vi "Autonomous Independent.vi"() -> ()   [LabVIEW 2012]
doc: "This VI is called when autonomous begins, and will automatically be terminated when autonomous ends. You can carry out timed or sensor driven robot movement independently without needing to return to the caller."
uses:
  AutoInstruction.ctl
  AutoEnum.ctl
  Robot Global Data.vi
  <vilib>/Rock Robotics/WPI/RobotDrive/WPI_RobotDriveArcadeDrive_Standard(NoSaturation).vi
panel:
  in  "Instructions":T1(array[cluster])
  in  "Instruction Sequence":T2(array[cluster])
  in  "AutoInstruction":T3
  in  "Default":T3[](array[typedef])
  in  "BackRight":T3[](array[typedef])
  in  "BackLeft":T3[](array[typedef])
  in  "FrontRight":T3[](array[typedef])
  in  "FrontLeft":T3[](array[typedef])
  out "AutoEnum":u16
  out "Current Movement, for debugging":T4 {"Y Joystick Value" scale=1.0..-1.0; "X Joystick Value" scale=-1.0..1.0}
  in  "Array of robot movements":T5(array[cluster]) {"Y Joystick Value" scale=1.0..-1.0; "X Joystick Value" scale=-1.0..1.0}
  # "Be sure to right-click and choose Data Operations>>Make Current Value default if you want to save the array values with the VI"
  # "REMEMBER TO SET AS DEFAULT"
  # "GLENN'S STUFF"
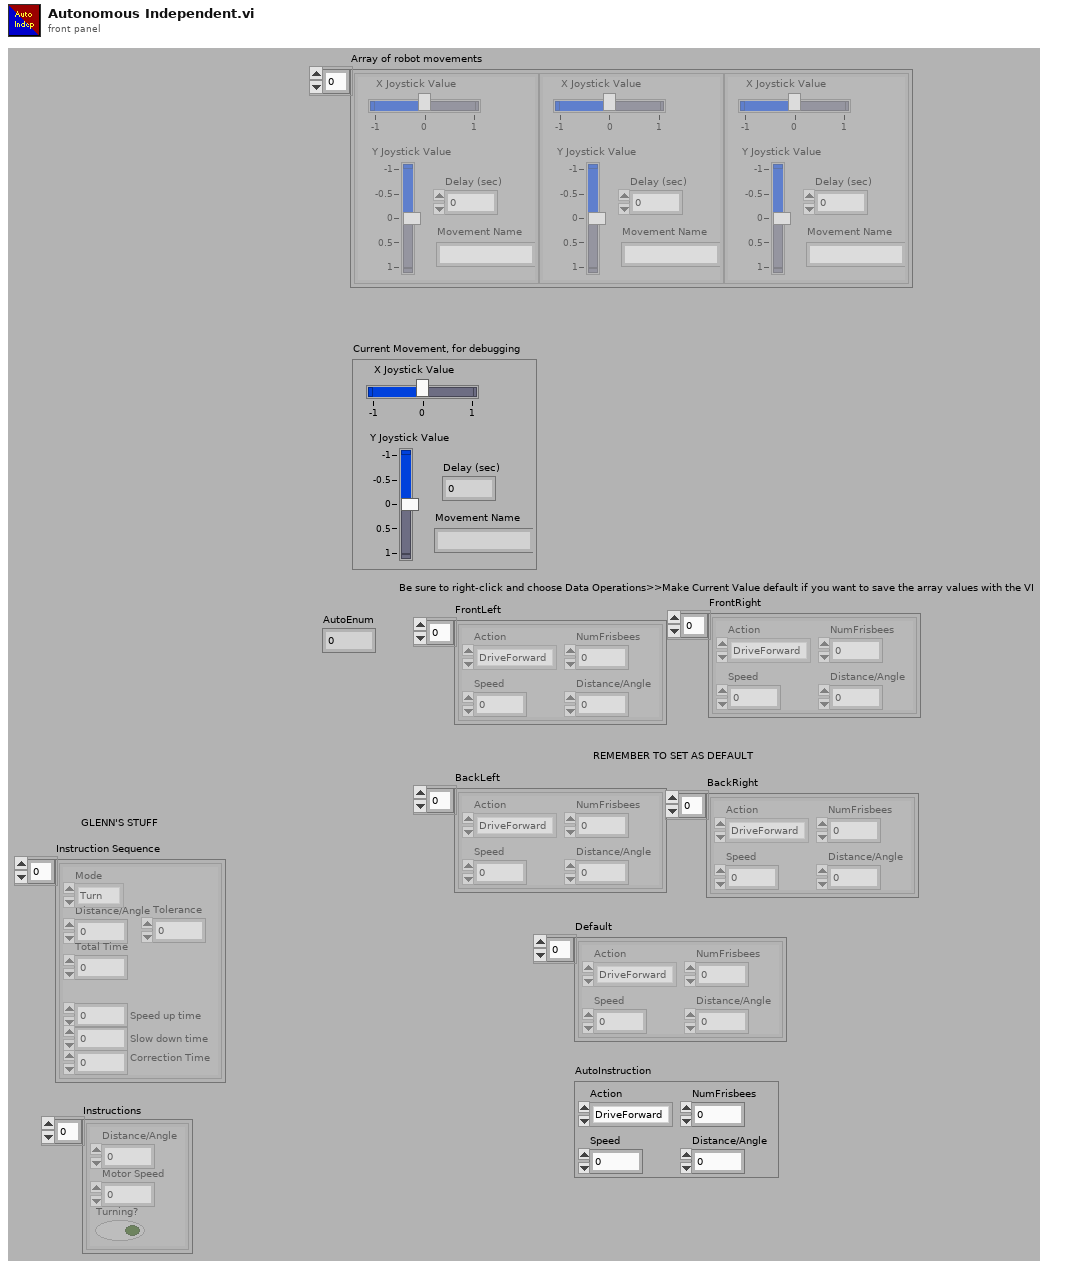
[diagram p1: front panel]
types:
  T1 = cluster{"Distance/Angle":dbl, "Motor Speed":dbl, "Turning?":bool}[]
  T2 = cluster{"Distance/Angle":dbl, "Tolerance":dbl, "Total Time":dbl, "Mode":enum16{"Turn", "Drive"}, "Correction Time":dbl, "Speed up time":dbl, "Slow down time":dbl}[]
  T3 = typedef "AutoInstruction.ctl" = cluster{"Distance/Angle":dbl, "Speed":dbl, "Action":enum16{"DriveForward", "Turn", "Aim", "Shoot"}, "NumFrisbees":i32}
  T4 = cluster{"X Joystick Value":dbl, "Y Joystick Value":dbl, "Delay (sec)":dbl, "Movement Name":string}
  T5 = cluster{"X Joystick Value":dbl, "Y Joystick Value":dbl, "Delay (sec)":dbl, "Movement Name":string}[]
  T6 = typedef "AutoEnum.ctl" = enum16{"Disabled", "BackRight", "BackLeft", "CloseRight", "CloseLeft"}
  T7 = typedef "WPI_EncoderDevRef.ctl" = cluster{"DevStatus":errorcluster, "EncoderIndex":T8, "CounterIndex":T9, "DistancePerCount":dbl, "Decoding Type":T10}
  T8 = typedef "FPGA_EncoderIdx.ctl" = enum8{"Enc 0", "Enc 1", "Enc 2", "Enc 3", "Invalid"}
  T9 = typedef "FPGA_CounterCtrSystemIndex.ctl" = enum8{"Ctr 0", "Ctr 1", "Ctr 2", "Ctr 3", "Ctr 4", "Ctr 5", "Ctr 6", "Ctr 7", "Invalid"}
  T10 = typedef "WPI_EncoderType.ctl" = enum16{"1x", "2x", "4x"}
  T11 = typedef "WPI_JoystickDevRef.ctl" = cluster{"Device":T12}
  T12 = typedef "WPI_JoystickDeviceEnum.ctl" = enum16{"USB 1", "USB 2", "USB 3", "USB 4", "Kinect 1", "Kinect 2"}
  T13 = cluster{"axis 1 (x)":dbl, "axis 2 (y)":dbl, "axis 3 (throttle)":dbl, "axis 4":dbl, "axis 5":dbl, "axis 6":dbl}
  T14 = typedef "WPI_GyroDevRef.ctl" = cluster{"DevStatus":errorcluster, "Analog Module":T15, "Analog Channel":T16, "Offset":dbl, "Gain (VoltsPerDegree/Second)":dbl}
  T15 = typedef "FPGA_TypedefAnalogModule.ctl" = enum16{"Analog Module 1", "Analog Module 2"}
  T16 = typedef "FPGA_AIChannel.ctl" = enum8{"AI 1", "AI 2", "AI 3", "AI 4", "AI 5", "AI 6", "AI 7", "AI 8", "Invalid"}
  T17 = typedef "WPI_RobotDriveDevRef.ctl" = cluster{"DevStatus":errorcluster, "Motors[]":T18[], "Square Inputs":bool, "Max Output":dbl, "Isochronous":bool}
  T18 = typedef "WPI_MotorControlDeviceRef.ctl" = cluster{"DeviceStatus":errorcluster, "Type":enum16{"PWM", "CAN"}, "PWM":cluster{"Digital Module":T19, "PWM Channel":T20, "DeadBand":T21}, "CAN":cluster{"Device Number":u8, "Control Mode":T22, "Semaphore":T23, "Max Vout":dbl}, "Invert":bool, "TransformRef":T24, "InvTransformRef":T24}
  T19 = typedef "FPGA_TypedefDigitalModule.ctl" = enum16{"Digital Module 1", "Digital Module 2"}
  T20 = typedef "FPGA_DIOPWMChannel.ctl" = enum8{"PWM 1", "PWM 2", "PWM 3", "PWM 4", "PWM 5", "PWM 6", "PWM 7", "PWM 8", "PWM 9", "PWM 10", "Invalid"}
  T21 = typedef "WPI_PWMDeadband.ctl" = cluster{"Name":string, "maxPositivePwm":i32, "minPositivePwm":i32, "centerPwm":i32, "maxNegativePwm":i32, "minNegativePwm":i32, "angularRange":u16}
  T22 = typedef "WPI_CANJaguar_ControlMode.ctl" = enum8{"Percent VBus", "Current", "Speed", "Position", "Voltage"}
  T23 = typedef "Semaphore RefNum" = refnum<k1>
  T24 = typedef "WPI_PWMTransform_ConPane.ctl" = refnum<vi>
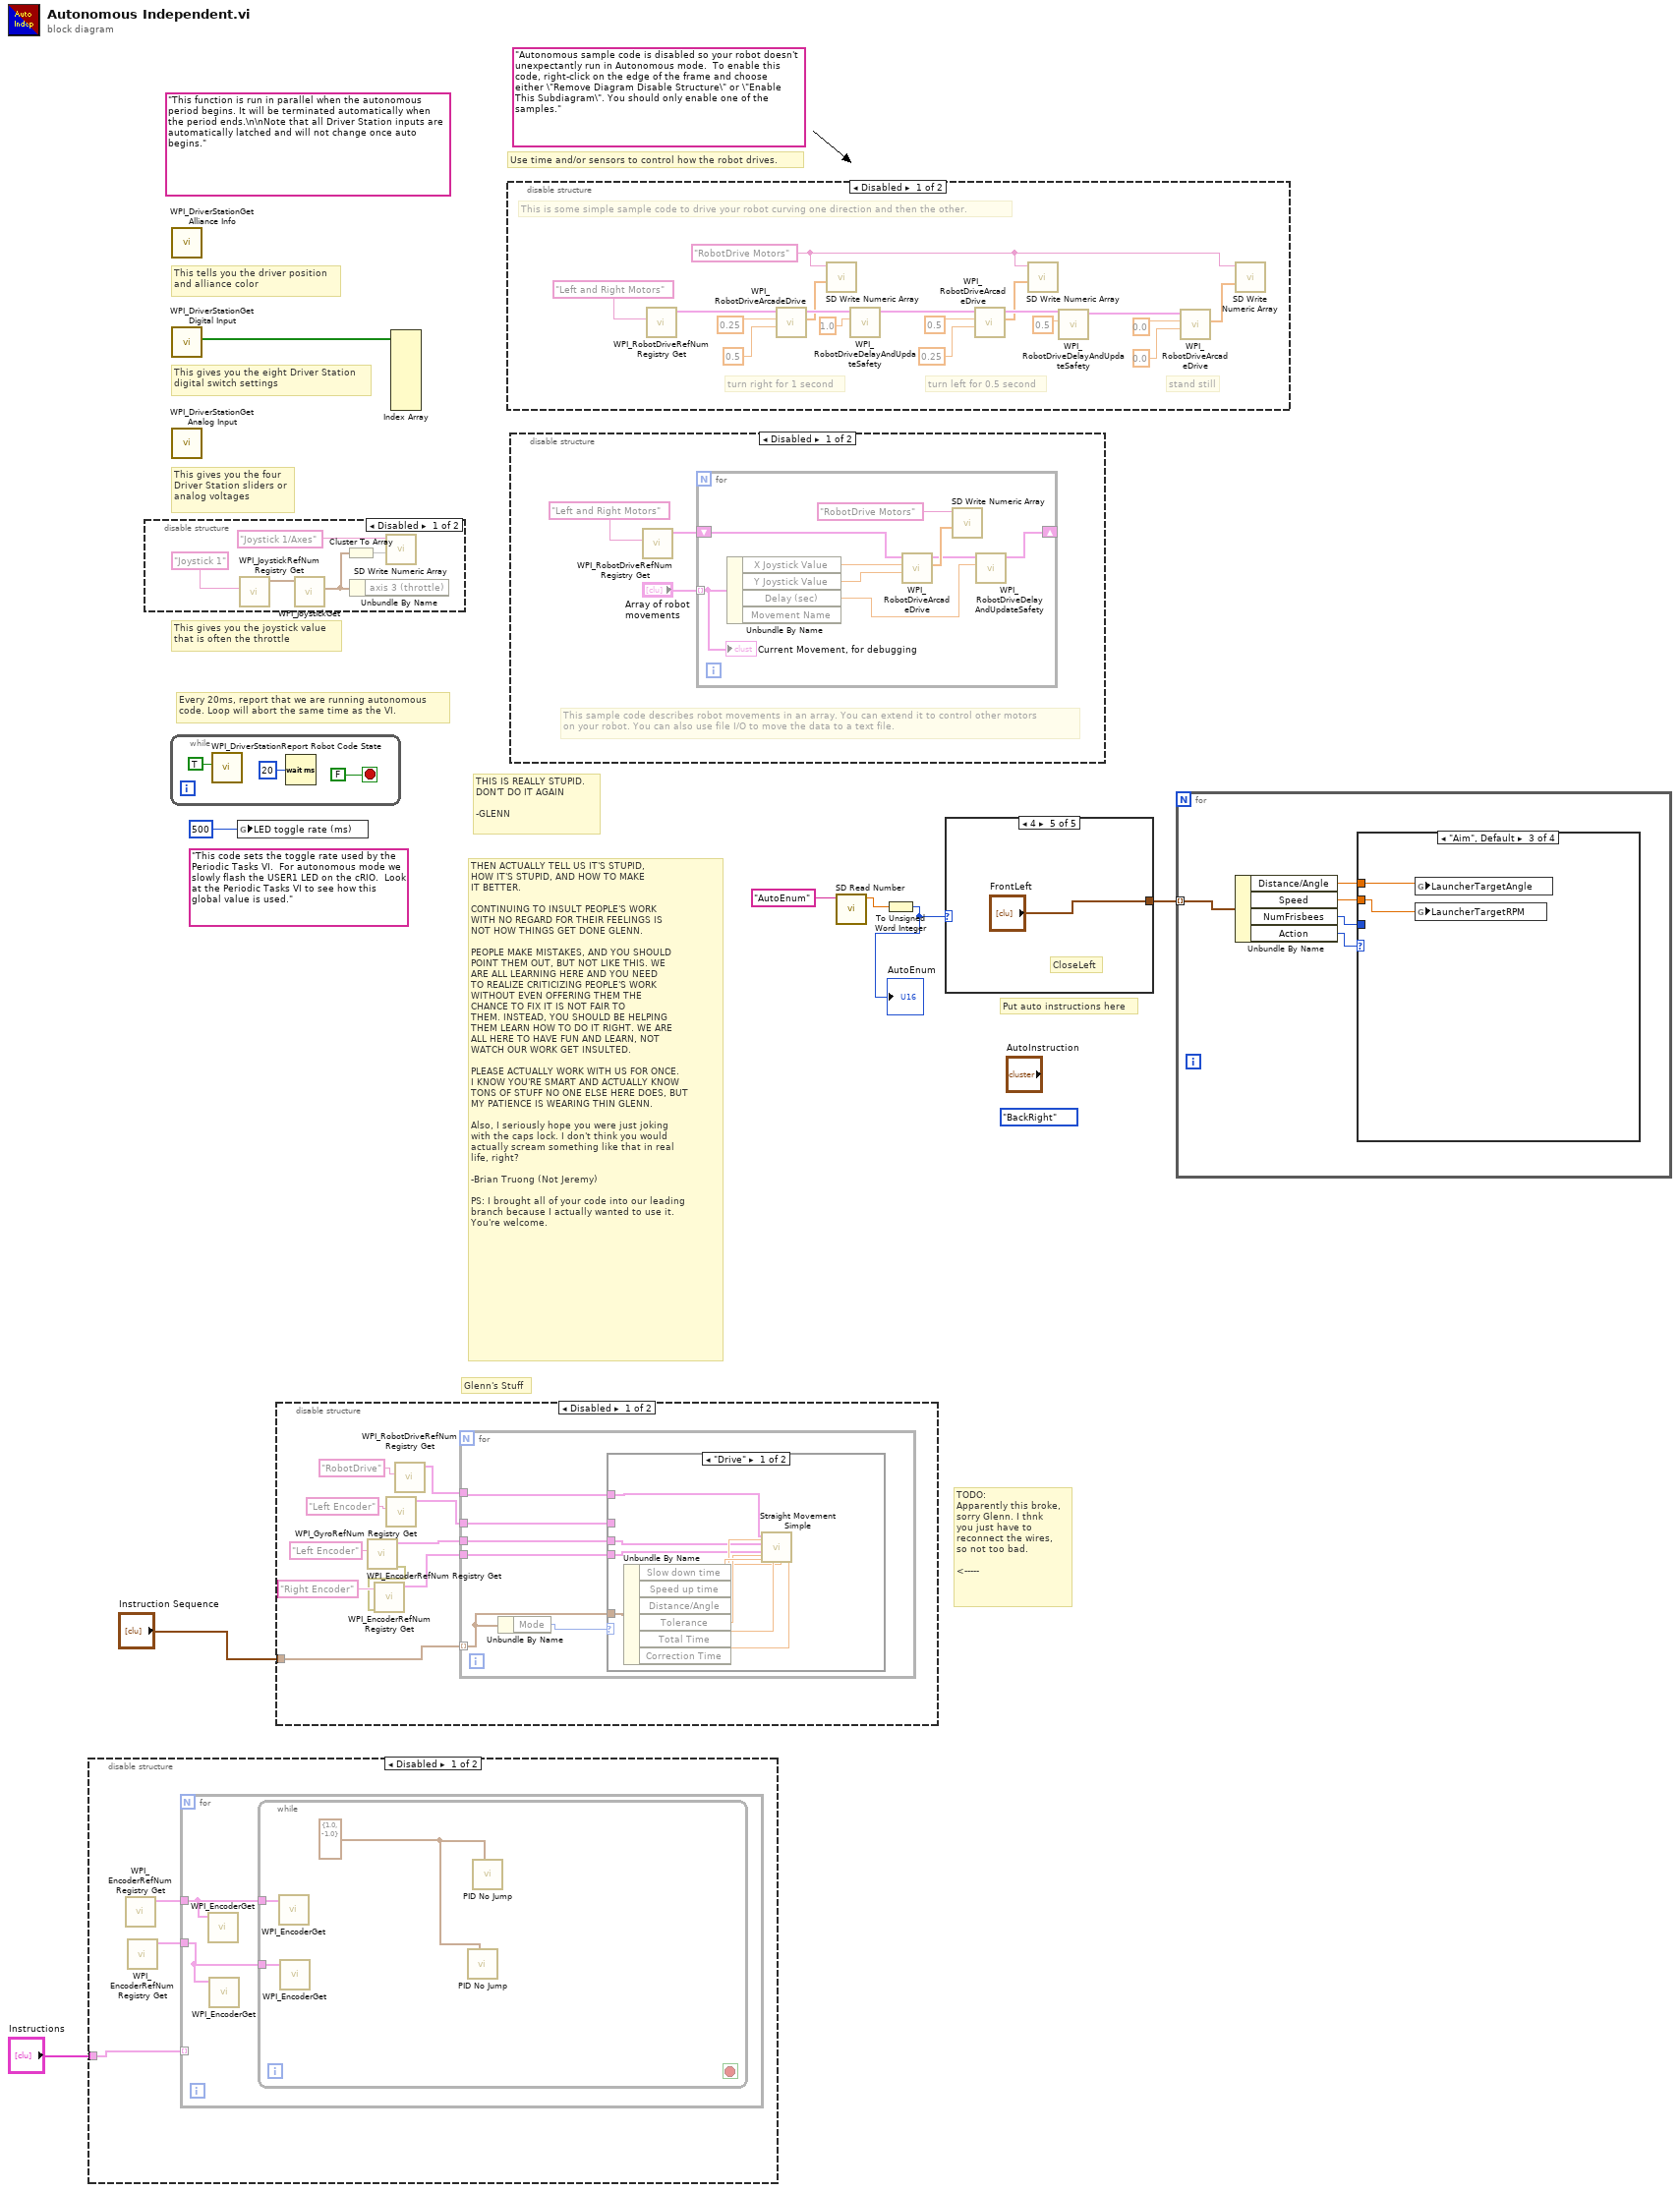
[diagram p0: block diagram]
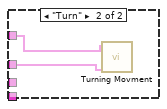
[diagram p4: hidden frame]
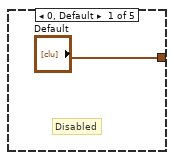
[diagram p6: hidden frame]
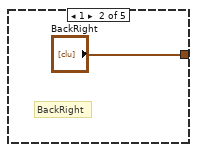
[diagram p7: hidden frame]
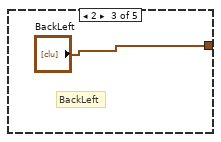
[diagram p8: hidden frame]
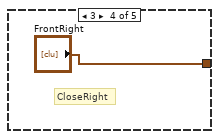
[diagram p9: hidden frame]
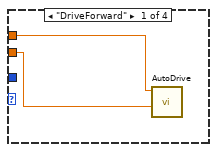
[diagram p10: hidden frame]
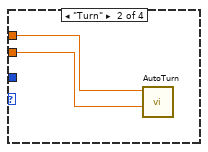
[diagram p11: hidden frame]
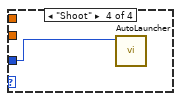
[diagram p12: hidden frame]
diagram:
  (unwired) AutoEnum."BackRight" ("AutoEnum")
  (unwired) "This code sets the toggle rate used by the Periodic Tasks VI.  For autonomous mode we slowly flash the USER1 LED on the cRIO.  Look at the Periodic Tasks VI to see how this global value is used."
  (unwired) "Autonomous sample code is disabled so your robot doesn't unexpectantly run in Autonomous mode.  To enable this code, right-click on the edge of the frame and choose either \"Remove Diagram Disable Structure\" or \"Enable This Subdiagram\". You should only enable one of the samples."
  (unwired) "This function is run in parallel when the autonomous period begins. It will be terminated automatically when the period ends.\n\nNote that all Driver Station inputs are automatically latched and will not change once auto begins."
  # "TODO:\nApparently this broke,\nsorry Glenn. I thnk\nyou just have to\nreconnect the wires,\nso not too bad.\n\n<-----"
  # "Glenn's Stuff"
  # "THEN ACTUALLY TELL US IT'S STUPID,\nHOW IT'S STUPID, AND HOW TO MAKE\nIT BETTER.\n\nCONTINUING TO INSULT PEOPLE'S WORK\nWITH NO REGARD FOR THEIR FEELINGS IS\nNOT HOW THINGS GET DONE GLENN.\n\nPEOPLE MAKE MISTAKES, AND YOU SHOULD\nPOINT THEM OUT, BUT NOT LIKE THIS. WE\nARE ALL LEARNING HERE AND YOU NEED\nTO REALIZE CRITICIZING PEOPLE'S WORK\nWITHOUT EVEN OFFERING THEM THE\nCHANCE TO FIX IT IS NOT FAIR TO\nTHEM. INSTEAD, YOU SHOULD BE HELPING\nTHEM LEARN HOW TO DO IT RIGHT. WE ARE\nALL HERE TO HAVE FUN AND LEARN, NOT\nWATCH OUR WORK GET INSULTED.\n\nPLEASE ACTUALLY WORK WITH US FOR ONCE.\nI KNOW YOU'RE SMART AND ACTUALLY KNOW\nTONS OF STUFF NO ONE ELSE HERE DOES, BUT\nMY PATIENCE IS WEARING THIN GLENN.\n\nAlso, I seriously hope you were just joking\nwith the caps lock. I don't think you would\nactually scream something like that in real\nlife, right?\n\n-Brian Truong (Not Jeremy)\n\nPS: I brought all of your code into our leading\nbranch because I actually wanted to use it.\nYou're welcome."
  # "THIS IS REALLY STUPID.\nDON'T DO IT AGAIN\n\n-GLENN"
  # "Put auto instructions here"
  # "Every 20ms, report that we are running autonomous\ncode. Loop will abort the same time as the VI."
  # "This gives you the joystick value\nthat is often the throttle"
  # "Use time and/or sensors to control how the robot drives."
  # "This tells you the driver position\nand alliance color"
  # "This gives you the eight Driver Station\ndigital switch settings"
  # "This gives you the four\nDriver Station sliders or\nanalog voltages"
  n1 = disable-structure shown="Disabled" {
    disable-tunnel: "Instructions" -> [w9 _]
    frame Disabled {
      n2 = call <vilib>:"WPI_EncoderRefNum Registry Get.vi"() -> ("EncoderDevRef"=w11:T7)  [unwired: 10 in, 1 out]
      n3 = call <vilib>:"WPI_EncoderRefNum Registry Get.vi"() -> ("EncoderDevRef"=w10:T7)  [unwired: 10 in, 1 out]
      n4 = for {
        tunnel: w11 -> [w13]
        tunnel: w10 -> [w12]
        tunnel: w9 -> [_] mode=indexing
        n5 = call <vilib>:"WPI_EncoderGet.vi"("EncoderDevRef"=w13) -> ()  [unwired: 5 in, 6 out]
        n6 = call <vilib>:"WPI_EncoderGet.vi"("EncoderDevRef"=w12) -> ()  [unwired: 5 in, 6 out]
        n7 = while {
          tunnel: w13 -> [w15]
          tunnel: w12 -> [w16]
          stop <- _ stop-if-true
          w14 = cluster{"output high":dbl, "output low":dbl} {"output high"=1.0, "output low"=-1.0} ("output range")
          n8 = call <vilib>:"WPI_EncoderGet.vi"("EncoderDevRef"=w15) -> ()  [unwired: 5 in, 6 out]
          n9 = call <vilib>:"WPI_EncoderGet.vi"("EncoderDevRef"=w16) -> ()  [unwired: 5 in, 6 out]
          n10 = call "PID No Jump.vi"("output range"=w14) -> ()  [unwired: 10 in, 1 out]
          n11 = call "PID No Jump.vi"("output range"=w14) -> ()  [unwired: 10 in, 1 out]
        }
      }
    }
    frame Enabled {
    }
  }
  n12 = disable-structure shown="Disabled" {
    frame Disabled {
      n13 = call <vilib>:"WPI_JoystickRefNum Registry Get.vi"("refnum name"="Joystick 1") -> ("JoystickDevRef"=w20:T11)  [unwired: 1 in, 9 out]
      n14 = call <vilib>:"WPI_JoystickGet.vi"("JoystickDevRef"=w20) -> ("Axes"=w18:T13)  [unwired: 1 in, 5 out]
      n15 = Cluster To Array(cluster=w18) -> (array=w19:dbl[])
      n16 = Unbundle By Name(w18) -> ()  [unwired: 1 out]
      n17 = call <vilib>:"SD Write Numeric Array.vi"("Numeric Array"=w19, "Name"="Joystick 1/Axes") -> ()  [unwired: 8 in, 2 out]
    }
    frame Enabled {
    }
  }
  n18 = while {
    stop <- FALSE stop-if-true
    n19 = call <vilib>:"WPI_DriverStationReport Robot Code State.vi"("Autonomous"=TRUE) -> ()  [unwired: 10 in, 1 out]
    n20 = Wait (ms)(milliseconds to wait=u32 20) -> ()  [unwired: 1 out]
  }
  n21 = call <vilib>:"WPI_DriverStationGet Alliance Info.vi"() -> ()  [unwired: 12 out]
  n22 = call <vilib>:"WPI_DriverStationGet Digital Input.vi"() -> ("Driver Station Digital Input (1-8)"=w8:bool[])  [unwired: 11 out]
  n23 = call <vilib>:"WPI_DriverStationGet Analog Input.vi"() -> ()  [unwired: 12 out]
  n24 = global write "Robot Global Data.vi" "LED toggle rate (ms)"(u32 500 ("LED ms toggle rate")) -> ()
  n25 = disable-structure shown="Disabled" {
    disable-tunnel: "Instruction Sequence" -> [w34 _]
    frame Disabled {
      n26 = call <vilib>:"WPI_EncoderRefNum Registry Get.vi"("refnum name"="Left Encoder") -> ("error out"=w25:errorcluster, "EncoderDevRef"=w31:T7)  [unwired: 9 in]
      n27 = call <vilib>:"WPI_EncoderRefNum Registry Get.vi"("error in (no error)"=w25, "refnum name"="Right Encoder") -> ("EncoderDevRef"=w30:T7)  [unwired: 8 in, 1 out]
      n28 = call <vilib>:"WPI_GyroRefNum Registry Get.vi"("refnum name"="Left Encoder") -> ("GyroDevRef"=w32:T14)  [unwired: 9 in, 1 out]
      n29 = call <vilib>:"WPI_RobotDriveRefNum Registry Get.vi"("refnum name"="RobotDrive") -> ("RobotDriveDevRef"=w33:T17)  [unwired: 9 in, 1 out]
      n30 = for {
        tunnel: w34 -> [w39] mode=indexing
        tunnel: w33 -> [w38]
        tunnel: w32 -> [w37]
        tunnel: w31 -> [w36]
        tunnel: w30 -> [w35]
        n31 = Unbundle By Name(w39) -> ("Mode"=w40:enum16{"Turn", "Drive"})
        n32 = case shown="\"Drive\"" w40 {
          tunnel: w39 -> [w50 _]
          tunnel: w38 -> [w43 w52]
          tunnel: w37 -> [_ w51]
          tunnel: w36 -> [w42 _]
          tunnel: w35 -> [w41 _]
          frame "Drive" {
            n33 = Unbundle By Name(w50) -> ("Slow down time"=w45:dbl, "Speed up time"=w44:dbl, "Distance/Angle"=w49:dbl, "Tolerance"=w48:dbl, "Total Time"=w47:dbl, "Correction Time"=w46:dbl)
            n34 = call "Straight Movement Simple.vi"(0:w46, 4:w48, 5:w45, 6:w47, 7:w44, 8:w49, "EncoderDevRef"=w41, "EncoderDevRef 2"=w42, "RobotDriveDevRef"=w43) -> ()  [unwired: 2 in, 1 out]
          }
          frame "Turn" {
            n35 = call "Turning Movment.vi"("GyroDevRef"=w51, "RobotDriveDevRef"=w52) -> ()  [unwired: 9 in, 1 out]
          }
        }
      }
    }
    frame Enabled {
    }
  }
  n36 = Index Array(array=w8) -> ()  [unwired: 8 in, 8 out]
  n37 = disable-structure shown="Disabled" {
    frame Disabled {
      w53 = "RobotDrive Motors" ("Name")
      # "This is some simple sample code to drive your robot curving one direction and then the other."
      # "stand still"
      # "turn left for 0.5 second"
      # "turn right for 1 second"
      n38 = call <vilib>:"WPI_RobotDriveRefNum Registry Get.vi"("refnum name"="Left and Right Motors") -> ("RobotDriveDevRef"=w57:T17)  [unwired: 1 in, 9 out]
      n39 = call-poly <vilib>:"WPI_RobotDriveArcadeDrive.vi"("Y axis value"=0.5 ("X axis value"), "X axis value"=0.25, "RobotDriveDevRef"=w57) -> ("Motor Values"=w56:dbl[], "RobotDriveDevRef"=w64:T17)  [unwired: 1 in, 6 out]
      n40 = call <vilib>:"SD Write Numeric Array.vi"("Numeric Array"=w56, "Name"=w53) -> ()  [unwired: 8 in, 2 out]
      n41 = call <vilib>:"WPI_RobotDriveDelayAndUpdateSafety.vi"("Delay (s)"=1.0, "RobotDriveDevRef"=w64) -> ("RobotDriveDevRef 2"=w63:T17)  [unwired: 8 in, 1 out]
      n42 = call-poly <vilib>:"WPI_RobotDriveArcadeDrive.vi"("Y axis value"=0.25 ("X axis value"), "X axis value"=0.5, "RobotDriveDevRef"=w63) -> ("Motor Values"=w55:dbl[], "RobotDriveDevRef"=w62:T17)  [unwired: 1 in, 6 out]
      n43 = call <vilib>:"SD Write Numeric Array.vi"("Numeric Array"=w55, "Name"=w53) -> ()  [unwired: 8 in, 2 out]
      n44 = call <vilib>:"WPI_RobotDriveDelayAndUpdateSafety.vi"("Delay (s)"=0.5, "RobotDriveDevRef"=w62) -> ("RobotDriveDevRef 2"=w61:T17)  [unwired: 8 in, 1 out]
      n45 = call-poly <vilib>:"WPI_RobotDriveArcadeDrive.vi"("Y axis value"=0.0 ("X axis value"), "X axis value"=0.0, "RobotDriveDevRef"=w61) -> ("Motor Values"=w54:dbl[])  [unwired: 1 in, 7 out]
      n46 = call <vilib>:"SD Write Numeric Array.vi"("Numeric Array"=w54, "Name"=w53) -> ()  [unwired: 8 in, 2 out]
    }
    frame Enabled {
    }
  }
  n47 = disable-structure shown="Disabled" {
    frame Disabled {
      # "This sample code describes robot movements in an array. You can extend it to control other motors\non your robot. You can also use file I/O to move the data to a text file."
      n48 = call <vilib>:"WPI_RobotDriveRefNum Registry Get.vi"("refnum name"="Left and Right Motors") -> ("RobotDriveDevRef"=w72:T17)  [unwired: 1 in, 9 out]
      n49 = for {
        shift-right: [w78] -> _
        shift-left: w72 -> [w79]
        tunnel: "Array of robot movements" -> [w74] mode=indexing
        n50 = Unbundle By Name(w74) -> ("X Joystick Value"=w77:dbl, "Y Joystick Value"=w76:dbl, "Delay (sec)"=w75:dbl)  [unwired: 1 out]
        n51 = call-poly <vilib>:"WPI_RobotDriveArcadeDrive.vi"("Y axis value"=w76, "X axis value"=w77, "RobotDriveDevRef"=w79) -> ("Motor Values"=w81:dbl[], "RobotDriveDevRef"=w80:T17)  [unwired: 1 in, 6 out]
        n52 = call <vilib>:"SD Write Numeric Array.vi"("Numeric Array"=w81, "Name"="RobotDrive Motors") -> ()  [unwired: 8 in, 2 out]
        n53 = call <vilib>:"WPI_RobotDriveDelayAndUpdateSafety.vi"("Delay (s)"=w75, "RobotDriveDevRef"=w80) -> ("RobotDriveDevRef 2"=w78:T17)  [unwired: 8 in, 1 out]
        "Current Movement, for debugging" <- w74
      }
    }
    frame Enabled {
    }
  }
  n54 = call <vilib>:"SD Read Number.vi"("Name"="AutoEnum") -> ("Numeric"=w5:dbl)  [unwired: 8 in, 2 out]
  n55 = To Unsigned Word Integer(number=w5) -> (unsigned 16bit integer=w4:u16)
  "AutoEnum" <- w4
  n56 = case shown="4" w4 {
    tunnel: ["Default" "BackRight" "BackLeft" "FrontRight" "FrontLeft"] -> w3
    frame 0, Default {
      # "Disabled"
    }
    frame 1 {
      # "BackRight"
    }
    frame 2 {
      # "BackLeft"
    }
    frame 3 {
      # "CloseRight"
    }
    frame 4 {
      # "CloseLeft"
    }
  }
  n57 = for {
    tunnel: w3 -> [w92] mode=indexing
    n58 = Unbundle By Name(w92) -> ("Distance/Angle"=w91:dbl, "Speed"=w90:dbl, "NumFrisbees"=w88:i32, "Action"=w89:enum16{"DriveForward", "Turn", "Aim", "Shoot"})
    n59 = case shown="\"Aim\", Default" w89 {
      tunnel: w91 -> [w94 w96 w98 _]
      tunnel: w90 -> [w93 w95 w97 _]
      tunnel: w88 -> [_ _ _ w99]
      frame "DriveForward" {
        n60 = call "AutoDrive.vi"("Steady Val"=w93, "Distance to travel (inches)"=w94) -> ()  [unwired: 10 in]
      }
      frame "Turn" {
        n61 = call "AutoTurn.vi"("Steady Val"=w95, "Degrees to turn"=w96) -> ()  [unwired: 10 in]
      }
      frame "Aim", Default {
        n62 = global write "Robot Global Data.vi" "LauncherTargetAngle"(w98) -> ()
        n63 = global write "Robot Global Data.vi" "LauncherTargetRPM"(w97) -> ()
      }
      frame "Shoot" {
        n64 = call "AutoLauncher.vi"("# Frisbees"=w99) -> ()  [unwired: 11 in]
      }
    }
  }
